vi "Converting Ascii strings to Hex strings.vi"(11 "result string":string) -> (3 "Chaîne":string)   [LabVIEW 2020, in "Library Commun.lvlib"]
uses:
  Library Commun.lvlib
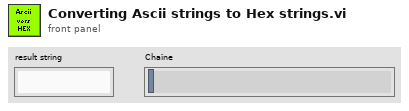
[diagram p1: front panel]
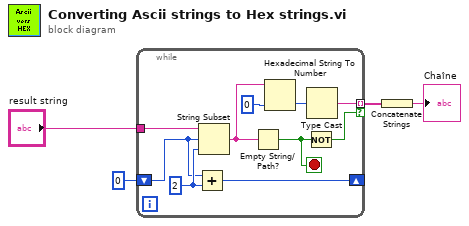
[diagram p0: block diagram]
diagram:
  n1 = while {
    tunnel: [w11] -> w1 mode=indexing if=w9
    shift-right: [w6] -> _
    shift-left: 0 ("longueur (reste)") -> [w7]
    tunnel: "result string" -> [w5]
    stop <- w10 stop-if-true
    w8 = 2 ("longueur (reste)")
    n2 = Add(x=w7, y=w8) -> (x+y=w6:i32)
    n3 = String Subset(string=w5, offset (0)=w7, length (rest)=w8) -> (substring=w12:string)
    n4 = Empty String/Path?(string/path=w12) -> (empty?=w10:bool)
    n5 = Hexadecimal String To Number(string=w12, default (0uL)=u8 0) -> (number=w13:u8)  [unwired: 1 in, 1 out]
    n6 = Not(x=w10) -> (.not. x?=w9:bool)
    n7 = Type Cast(x=w13) -> (*(type *) &x=w11:string)  [unwired: 1 in]
  }
  n8 = Concatenate Strings(w1) -> (→"Chaîne":string)
